vi "Val to angle left.vi"(11 "Sensor val":dbl) -> (3 "Left bending angle":dbl format="%_6f")   [LabVIEW 2019]
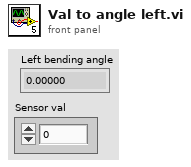
[diagram p1: front panel]
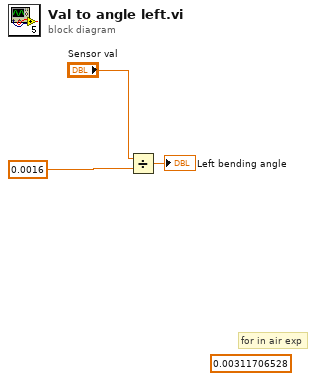
[diagram p0: block diagram]
diagram:
  (unwired) 0.00311706528
  # "for in air exp"
  n1 = Divide(x="Sensor val", y=0.0016) -> (x/y=→"Left bending angle":dbl)
